vi "Periodic Tasks1.vi"(8 "error in":errorcluster) -> ()   [LabVIEW 2015]
doc: "This VI runs in parallel to other tasks. It can contain as many user-defined periodic loops as you need. These can carry out PID or other sorts of timed response."
uses:
  <vilib>/Rock Robotics/WPI/Solenoid/WPI_SolenoidChannel.ctl
  <vilib>/Rock Robotics/SystemInterfaces/DIO/FPGA_DIOPWMChannel.ctl
  <vilib>/Rock Robotics/WPI/Solenoid/WPI_SolenoidValue.ctl
  <vilib>/Rock Robotics/WPI/Utilities/WPI_GetSetVariantRefNum.vi
  <vilib>/Rock Robotics/WPI/Solenoid/WPI_SolenoidOpenSingle.vi
  <vilib>/Rock Robotics/WPI/MotorControl/WPI_MotorControlOpen VictorSP.vi
  <vilib>/Rock Robotics/WPI/Solenoid/WPI_SolenoidSetEnum.vi
panel:
  out "Lift/lower 2":string
  out "Button 5":bool
  out "Button 4":bool
  out "Button 3":bool
  out "Button 2":bool
  out "Lift/lower 1":string
  out "Button 1":bool
  out "Compressor Monitoring?":bool
  in  "Solenoid Channel":T1
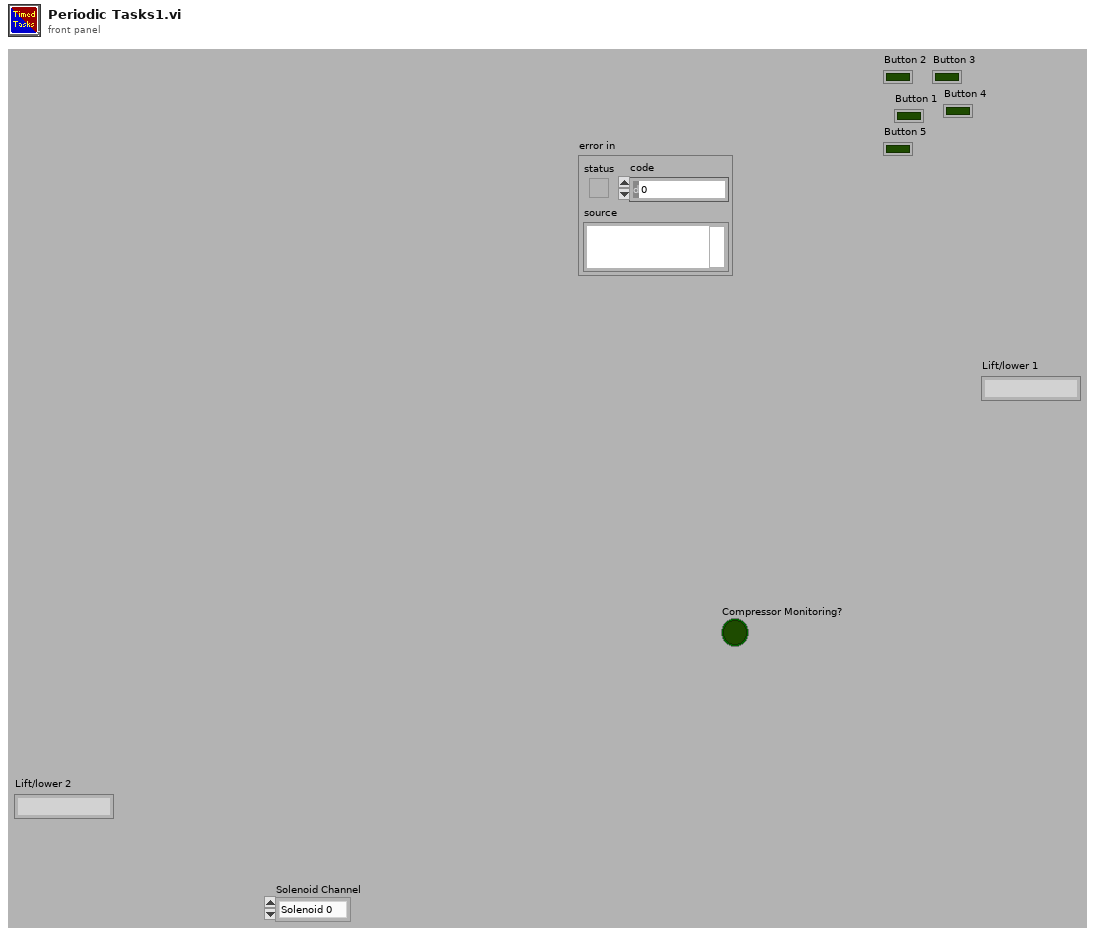
[diagram p1: front panel]
types:
  T1 = typedef "WPI_SolenoidChannel.ctl" = enum8{"Solenoid 0", "Solenoid 1", "Solenoid 2", "Solenoid 3", "Solenoid 4", "Solenoid 5", "Solenoid 6", "Solenoid 7", "Invalid"}
  T2 = typedef "FPGA_DIOPWMChannel.ctl" = enum8{"PWM 0", "PWM 1", "PWM 2", "PWM 3", "PWM 4", "PWM 5", "PWM 6", "PWM 7", "PWM 8", "PWM 9", "PWM MXP 0", "PWM MXP 1", "PWM MXP 2", "PWM MXP 3", "PWM MXP 4", "PWM MXP 5", "PWM MXP 6", "PWM MXP 7", "PWM MXP 8", "PWM MXP 9", "Invalid"}
  T3 = typedef "WPI_CompressorDevRef.ctl" = cluster{"DevStatus":errorcluster, "Pneumatics Control Module":u8}
  T4 = typedef "WPI_JoystickDevRef.ctl" = cluster{"Device":T5}
  T5 = typedef "WPI_JoystickDeviceEnum.ctl" = enum16{"USB 0", "USB 1", "USB 2", "USB 3", "USB 4", "USB 5"}
  T6 = typedef "WPI_RobotDriveDevRef.ctl" = cluster{"DevStatus":errorcluster, "Motors[]":T7[], "Square Inputs":bool, "Max Output":dbl}
  T7 = typedef "WPI_MotorControlDeviceRef.ctl" = cluster{"DeviceStatus":errorcluster, "Type":T8, "PWM":cluster{"PWM Channel":T2, "DeadBand":T9}, "CAN":cluster{"Device Number":u8, "Control Mode":T10, "Semaphore":T11, "Max Vout":dbl, "TalonSRX Control Mode":T12}, "Invert":bool}
  T8 = typedef "WPI_MotorControlType.ctl" = enum16{"PWM", "CAN", "CANTalonSRX"}
  T9 = typedef "WPI_PWMDeadband.ctl" = cluster{"Name":string, "maxPositivePwm":i32, "minPositivePwm":i32, "centerPwm":i32, "maxNegativePwm":i32, "minNegativePwm":i32, "angularRange":u16}
  T10 = typedef "WPI_CANJaguar_ControlMode.ctl" = enum8{"Percent VBus", "Current", "Speed", "Position", "Voltage"}
  T11 = typedef "Semaphore RefNum" = refnum<k1>
  T12 = typedef "WPI_CANTalonSRX_APIControlMode.ctl" = enum8{"Percent VBus", "Speed", "Position", "Slave", "Unchanged / Invalid", "Voltage Compensation", "Current", "Motion Profile"}
  T13 = typedef "WPI_SolenoidDevRef.ctl" = cluster{"DevStatus":errorcluster, "Pneumatics Control Module":u8, "Forward Solenoid Channel":T1, "Reverse Solenoid Channel":T1}
  T14 = cluster{"JoystickDevRef":T4, "RobotDriveDevRef":T6, "SolenoidDevRef":T13}
  T15 = typedef "WPI_SolenoidValue.ctl" = enum16{"Off", "On", "Forward", "Reverse"}
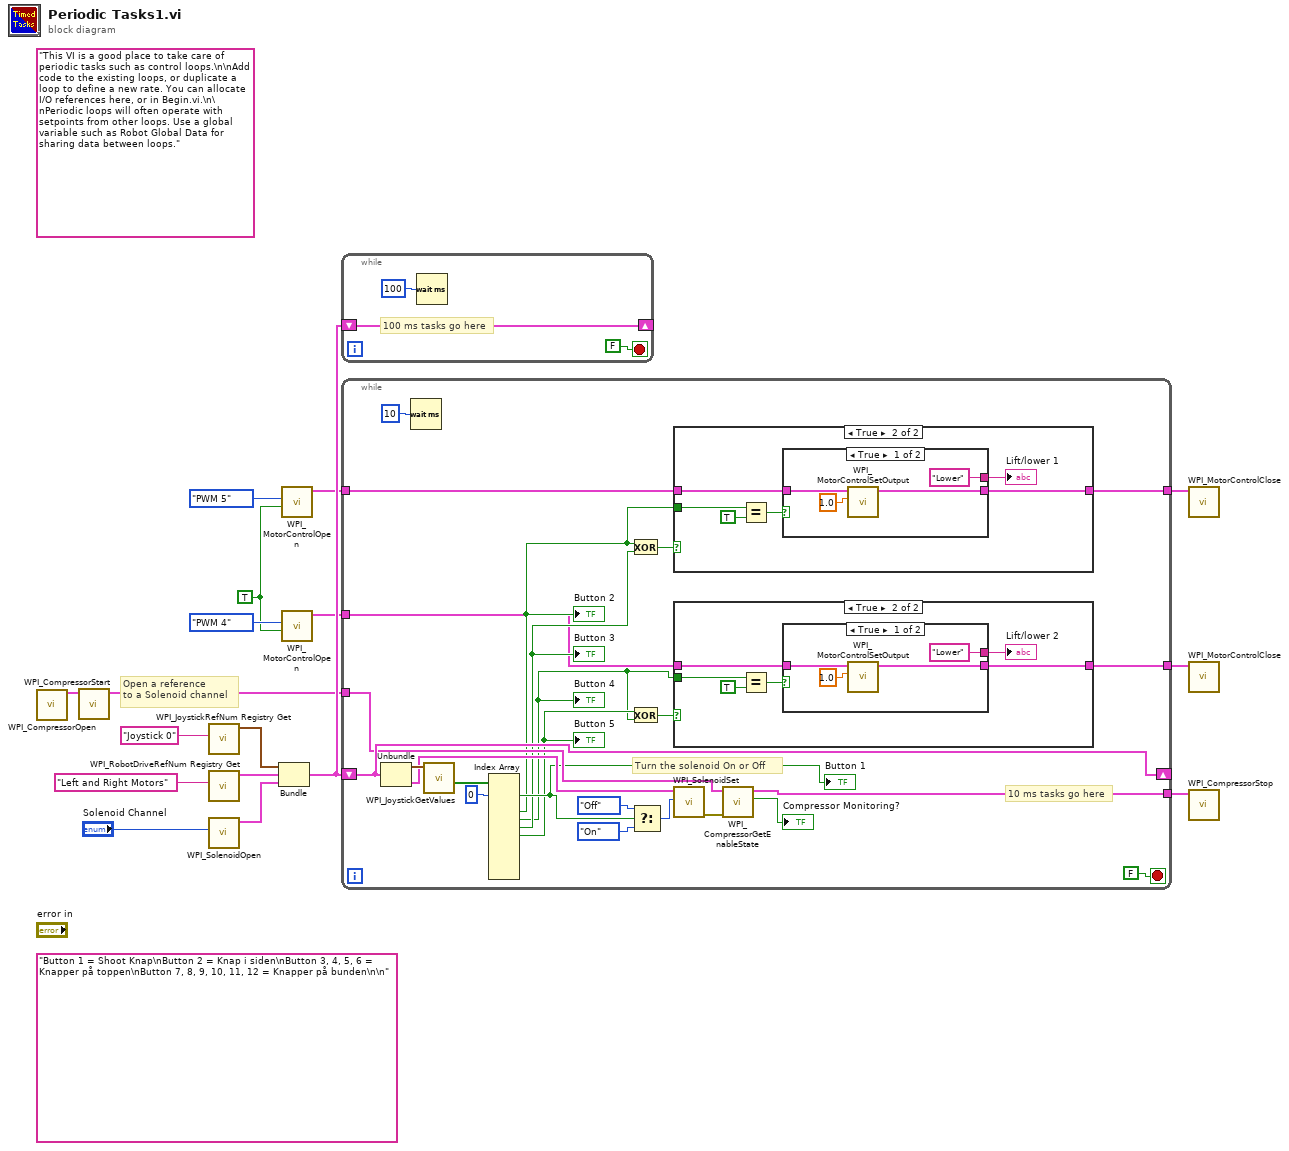
[diagram p0: block diagram]
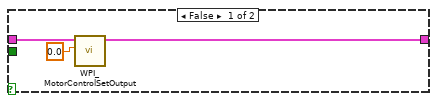
[diagram p2: hidden frame]
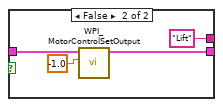
[diagram p3: hidden frame]
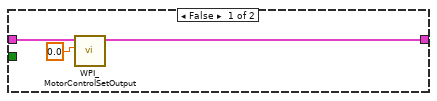
[diagram p4: hidden frame]
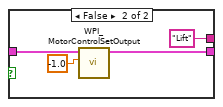
[diagram p5: hidden frame]
diagram:
  w1 = TRUE ("Eliminate Deadband")
  (unwired) "Button 1 = Shoot Knap\nButton 2 = Knap i siden\nButton 3, 4, 5, 6 = Knapper på toppen\nButton 7, 8, 9, 10, 11, 12 = Knapper på bunden\n\n"
  (unwired) "This VI is a good place to take care of periodic tasks such as control loops.\n\nAdd code to the existing loops, or duplicate a loop to define a new rate. You can allocate I/O references here, or in Begin.vi.\n\nPeriodic loops will often operate with setpoints from other loops. Use a global variable such as Robot Global Data for sharing data between loops."
  # "Open a reference \nto a Solenoid channel"
  n1 = call <vilib>:"WPI_CompressorOpen.vi"() -> ("CompressorDevRef"=w10:T3)  [unwired: 14 in, 1 out]
  n2 = call <vilib>:"WPI_CompressorStart.vi"("CompressorDevRef"=w10) -> ("CompressorDevRef"=w9:T3)  [unwired: 3 in, 7 out]
  n3 = call <vilib>:"WPI_JoystickRefNum Registry Get.vi"("refnum name"="Joystick 0") -> ("JoystickDevRef"=w15:T4)  [unwired: 1 in, 9 out]
  n4 = call <vilib>:"WPI_RobotDriveRefNum Registry Get.vi"("refnum name"="Left and Right Motors") -> ("RobotDriveDevRef"=w14:T6)  [unwired: 1 in, 9 out]
  n5 = call-poly <vilib>:"WPI_SolenoidOpen.vi"("Solenoid Channel"="Solenoid Channel") -> ("SolenoidDevRef"=w11:T13)  [unwired: 2 in, 8 out]
  n6 = Bundle("JoystickDevRef"=w15, "RobotDriveDevRef"=w14, "SolenoidDevRef"=w11) -> (w13:T14)  [unwired: 1 out]
  n7 = call-poly <vilib>:"WPI_MotorControlOpen.vi"("Eliminate Deadband"=w1, "PWM Channel"=FPGA_DIOPWMChannel."PWM 5") -> ("MotorControlDeviceRef"=w7:T7)  [unwired: 8 in, 1 out]
  n8 = call-poly <vilib>:"WPI_MotorControlOpen.vi"("Eliminate Deadband"=w1, "PWM Channel"=FPGA_DIOPWMChannel."PWM 4") -> ("MotorControlDeviceRef"=w3:T7)  [unwired: 8 in, 1 out]
  n9 = while {
    shift-right: [w18] -> _
    shift-left: w13 -> [w18]
    stop <- FALSE stop-if-true
    # "100 ms tasks go here"
    n10 = Wait (ms)(milliseconds to wait=u32 100) -> ()  [unwired: 1 out]
  }
  n11 = while {
    shift-right: [w43] -> _
    shift-left: w13 -> [w43]
    tunnel: w9 -> [w34]
    tunnel: [w33] -> w8
    tunnel: w7 -> [w29]
    tunnel: w3 -> [w24]
    tunnel: [w21] -> w4
    tunnel: [w28] -> w5
    stop <- FALSE stop-if-true
    # "10 ms tasks go here"
    # "Turn the solenoid On or Off"
    n12 = Unbundle(w43) -> ("JoystickDevRef"=w42:T4, "SolenoidDevRef"=w37:T13)  [unwired: 1 out]
    n13 = Wait (ms)(milliseconds to wait=u32 10) -> ()  [unwired: 1 out]
    n14 = call <vilib>:"WPI_JoystickGetValues.vi"("JoystickDevRef"=w42) -> ("Buttons"=w41:bool[])  [unwired: 6 in, 4 out]
    n15 = Index Array(array=w41, index #1=0 ("index")) -> (element #1=w31:bool, element #3=w25:bool, element #4=w23:bool, element #5=w27:bool, element #6=w30:bool)  [unwired: 10 in, 6 out]
    "Button 1" <- w31
    "Button 2" <- w25
    "Button 3" <- w27
    "Button 4" <- w23
    "Button 5" <- w30
    n16 = Exclusive Or(1:w27, 2:w25) -> (0:w26:bool)
    n17 = Exclusive Or(1:w23, 2:w30) -> (0:w22:bool)
    n18 = Select(t=WPI_SolenoidValue."Off" ("Value"), s=w31, f=WPI_SolenoidValue."On" ("Value")) -> (s? t:f=w38:T15)
    n19 = case shown="True" w26 {
      tunnel: w29 -> [w65 w71]
      tunnel: [w64 w69] -> w28
      tunnel: w25 -> [_ w68]
      frame False {
        n20 = call <vilib>:"WPI_MotorControlSetOutput.vi"("Output"=0.0, "MotorControlDevRef"=w65) -> ("MotorControlDevRef"=w64:T7)  [unwired: 7 in, 2 out]
      }
      frame True {
        n21 = Equal?(x=w68, y=TRUE) -> (x = y?=w66:bool)
        n22 = case shown="True" w66 {
          tunnel: [w73 w76] -> w69
          tunnel: ["Lower" "Lift"] -> w70
          tunnel: w71 -> [w74 w77]
          frame True {
            n23 = call <vilib>:"WPI_MotorControlSetOutput.vi"("Output"=1.0, "MotorControlDevRef"=w74) -> ("MotorControlDevRef"=w73:T7)  [unwired: 7 in, 2 out]
          }
          frame False {
            n24 = call <vilib>:"WPI_MotorControlSetOutput.vi"("Output"=-1.0, "MotorControlDevRef"=w77) -> ("MotorControlDevRef"=w76:T7)  [unwired: 7 in, 2 out]
          }
        }
        "Lift/lower 1" <- w70
      }
    }
    n25 = case shown="True" w22 {
      tunnel: w24 -> [w48 w54]
      tunnel: [w47 w52] -> w21
      tunnel: w23 -> [_ w51]
      frame False {
        n26 = call <vilib>:"WPI_MotorControlSetOutput.vi"("Output"=0.0, "MotorControlDevRef"=w48) -> ("MotorControlDevRef"=w47:T7)  [unwired: 7 in, 2 out]
      }
      frame True {
        n27 = Equal?(x=w51, y=TRUE) -> (x = y?=w49:bool)
        n28 = case shown="True" w49 {
          tunnel: [w56 w59] -> w52
          tunnel: ["Lower" "Lift"] -> w53
          tunnel: w54 -> [w57 w60]
          frame True {
            n29 = call <vilib>:"WPI_MotorControlSetOutput.vi"("Output"=1.0, "MotorControlDevRef"=w57) -> ("MotorControlDevRef"=w56:T7)  [unwired: 7 in, 2 out]
          }
          frame False {
            n30 = call <vilib>:"WPI_MotorControlSetOutput.vi"("Output"=-1.0, "MotorControlDevRef"=w60) -> ("MotorControlDevRef"=w59:T7)  [unwired: 7 in, 2 out]
          }
        }
        "Lift/lower 2" <- w53
      }
    }
    n31 = call-poly <vilib>:"WPI_SolenoidSet.vi"("Value"=w38, "SolenoidDevRef"=w37) -> ("error out"=w35:errorcluster)  [unwired: 1 in, 8 out]
    n32 = call <vilib>:"WPI_CompressorGetEnableState.vi"("error in (no error)"=w35, "CompressorDevRef"=w34) -> ("Enabled"=→"Compressor Monitoring?":bool, "CompressorDevRef"=w33:T3)  [unwired: 8 out]
  }
  n33 = call <vilib>:"WPI_MotorControlClose.vi"("MotorControlDevRef"=w5) -> ()  [unwired: 10 in, 1 out]
  n34 = call <vilib>:"WPI_MotorControlClose.vi"("MotorControlDevRef"=w4) -> ()  [unwired: 10 in, 1 out]
  n35 = call <vilib>:"WPI_CompressorStop.vi"("CompressorDevRef"=w8) -> ()  [unwired: 1 in, 10 out]
